vi "Dashboard Main_1366_768.vi"() -> ()   [LabVIEW 2020]
uses:
  <vilib>/Rock Robotics/WPI/ThirdParty/JAS_Junk/TrajLib/TypeDef/FieldDisp_ElementPicture.ctl
  <vilib>/event_ctls.llb/eventvkey.ctl
  <vilib>/Rock Robotics/WPI/ThirdParty/JAS_Junk/TrajLib/Rotation2d_CreateAngle.vi
  <vilib>/Rock Robotics/WPI/ThirdParty/JAS_Junk/TrajLib/Translation2d_Create.vi
  <vilib>/Rock Robotics/WPI/ThirdParty/JAS_Junk/TrajLib/VI/FieldDisp_Element_Rotate.vi
  <vilib>/Rock Robotics/WPI/ThirdParty/JAS_Junk/TrajLib/Conv_Meters_Inches.vi
  <vilib>/Rock Robotics/WPI/ThirdParty/JAS_Junk/TrajLib/Conv_Radians_Deg.vi
  <vilib>/Rock Robotics/WPI/Dashboard/WPI_DashboardLogging Global.vi
  <vilib>/Rock Robotics/Network Tables/NT Read Boolean.vi
  <vilib>/Rock Robotics/Network Tables/NT Write Boolean.vi
  <vilib>/Rock Robotics/Network Tables/NT Read Numeric Array.vi
  <vilib>/picture/pixmap.llb/Flatten Pixmap.vi
  <vilib>/picture/pictutil.llb/Create Mask.vi
  <vilib>/picture/picture.llb/Draw Flattened Pixmap.vi
  <vilib>/Rock Robotics/WPI/ThirdParty/JAS_Junk/TrajLib/Trajectory_Library.lvlib
panel:
  out "Popcorn Engaged":bool
  out "ROBOT":T1
  out "Camera Perf":string
  in  "Camera Settings":T2={"Frame Rate"=30, "Compression"=30, "Size"=1, "DB Camera Config"=FALSE} {"Frame Rate" scale=1.0..30.0; "Compression" scale=100.0..-1.0; "Size" items=["640x480", "320x240", "160x120"]}
  in  "TCP":refnum<k5>
  in  "Rec Mode":enum32{"Stop", "Record", "Playback"}(radio)
  out "Robot IP":string
  out "Image Message":string="Timeout in Camera Communications"
  in  "Dashboard Tab":T3(tab)
  out "MotorChart L":cluster{"Numeric":dbl, "Numeric":dbl}(graph)
  out "MotorSliders L":cluster{"MotorSlide1":dbl, "MotorSlide2":dbl} {"MotorSlide2" scale=-1.0..1.0 scale format="%#_2e"; "MotorSlide1" scale=-1.0..1.0 scale format="%#_2e"}
  out "MotorChart R":cluster{"Numeric":dbl, "Numeric":dbl}(graph)
  out "MotorSliders R":cluster{"MotorSlide1":dbl, "MotorSlide2":dbl} {"MotorSlide2" scale=-1.0..1.0 scale format="%#_2e"; "MotorSlide1" scale=-1.0..1.0 scale format="%#_2e"}
  out "To infinity and beyond?":string
  out "Climb Override":bool
  out "Climbing Stages":sgl(slide) scale=0.0..10.0 scale format="%#_6p"
  out "Reverse":bool
  out "Drive Mode":string
  out "Selected Auto":string
  in  "Select Auto":string(combo)="Select Autonomous ..."
  out "NT Connection":bool
  out "Mode":T4(ring)=enum."Auto Disabled"
  out "Right Camera Perf":cluster{"Bandwidth (Mbps)":dbl, "FPS":dbl}
  in  "ARE YOU READY TO RUMBLE":bool
  out "Lidar":dbl(knob) scale=0.0..10.0
  out "JS2 Z":dbl(slide) scale=-1.0..1.0 scale format="%#_2e"
  out "JS2 Graph":cluster{"X":dbl, "Y":dbl}[](graph)
  out "JS2 Buttons":T5
  out "JS1 Z":dbl(slide) scale=-1.0..1.0 scale format="%#_2e"
  out "JS1 Graph":cluster{"X":dbl, "Y":dbl}[](graph)
  out "JS1 Buttons":T5
  out "Wall!":bool
  out "Right April Tag Updated":bool
  out "Left April Tag Updated":bool
  out "Right Cam Connected":bool
  out "Left Cam Connected":bool
  out "Field Picture":picture
  out "Odom X Pos Ft":dbl format="%14.2f"
  out "Odom Y Pos Ft":dbl format="%14.2f"
  out "Odom Heading Deg":dbl format="%14.2f"
  in  "Shooter Demand":dbl
  out "Shooter Speed":dbl
  out "Shooter Speed Trend":T6(graph)
  out "Target Shooter Speed":dbl
  out "Motor Output":dbl
  in  "Dashboard Tab 2":T7(tab)
  out "Speed Chart Left":cluster{"Numeric":dbl, "Numeric":dbl}(graph)
  out "Speed Chart Right":cluster{"Numeric":dbl, "Numeric":dbl}(graph)
  in  "Dont Question it":bool
  out "Right Speed Demand":dbl
  out "Left Speed Demand":dbl
  out "Right Speed":dbl
  out "Left Speed":dbl
  out "Deviation Threshold 2":dbl
  out "Filter Height 2":dbl
  in  "Deviation Threshold":dbl
  in  "Filter Height":dbl
  out "Current Filter":T8={"Hue"={110.0, 142.0}, "Saturation"={0.0, 209.6394230769231}, "Value"={0.0, 105.16949152542372}} {"Value" scale=0.0..255.0; "Saturation" scale=0.0..255.0; "Hue" scale=0.0..255.0 scale format="%#_3g"}
  in  "New Filter":T8={"Hue"={110.0, 142.0}, "Saturation"={0.0, 209.6394230769231}, "Value"={0.0, 105.16949152542372}} {"Value" scale=0.0..255.0; "Saturation" scale=0.0..255.0; "Hue" scale=0.0..255.0 scale format="%#_3g"}
  in  "Update\nVision\nTuning":bool
  out "Bananas Engaged":bool
  in  "DONUT PRESS":bool
  out "Bandwidth (Mbps)":dbl
  out "FPS":dbl
  in  "Test Slider":dbl(slide) scale=0.0..100.0 scale format="%#_3g"
  in  "On/Off":bool caption="Solenoid"
  in  "Test Name":u16(ring) items=["Select the test to run..."]
  in  "Test Tree":string(tree)
  in  "Motor":cluster{"Value":dbl, "Enable":bool} {"Value" scale=-1.0..1.0 scale format="%#_3g"}
  out "Progress":T9 {"Test Progress" scale=0.0..100.0}
  in  "Rev/Fwd":cluster{"Forward":bool, "Reverse":bool}
  in  "Test Ring":u16(ring) items=["Monochrome", "Color"]
  in  "CheckList":i32(listbox)
  out "Tree":string(tree)
  out "Camera Image":T10(plugin-control)
  out "Background":bool
  in  "Camera Name":string(combo)="No Camera Selection"
  # "HW"
  # "Joysticks"
  # "Drive Motors"
  # "Front"
  # "Left"
  # "Right"
  # "Back"
  # "Right"
  # "Left"
  # "Speed D"
  # "Speed"
  # "DONUT PRESS"
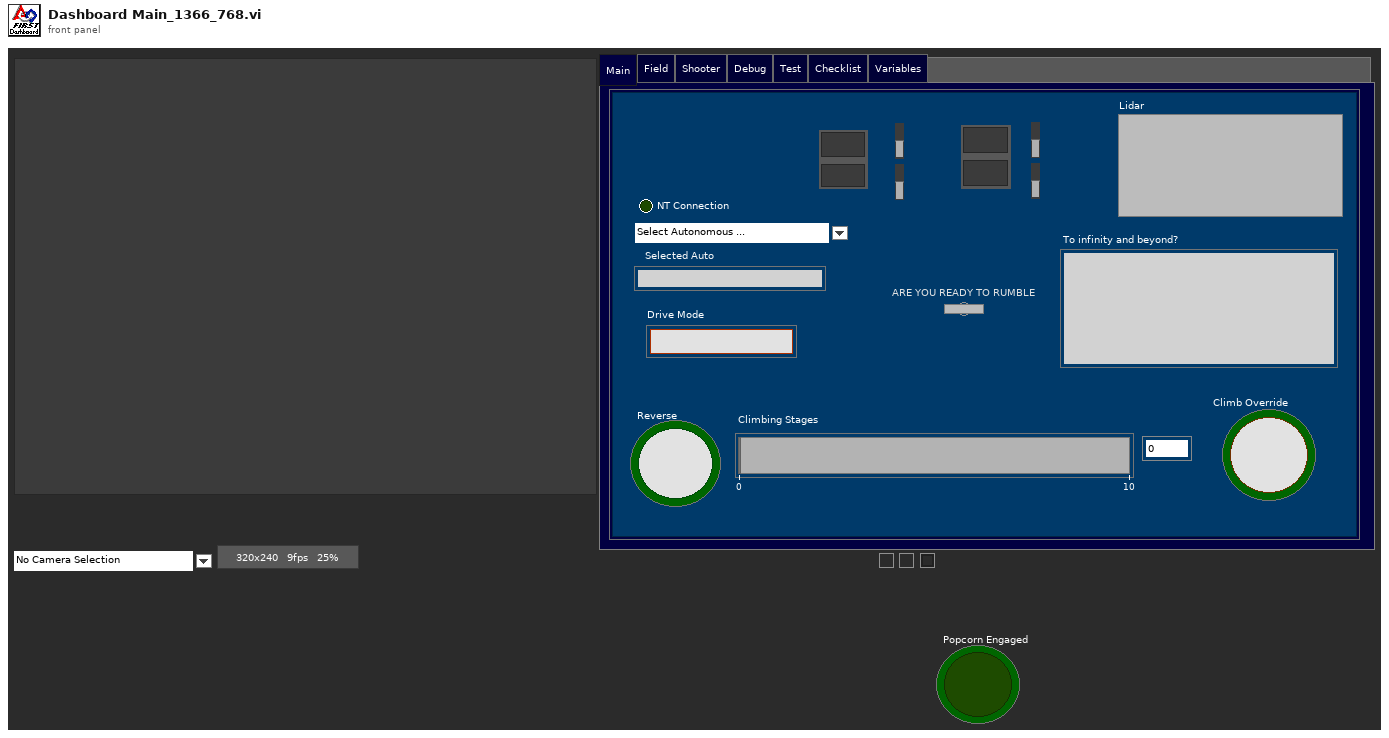
[diagram p1: front panel]
types:
  T1 = typedef "Trajectory_Library.lvlib/FieldDisp_ElementPicture.ctl" = picture
  T2 = cluster{"Frame Rate":i32, "Compression":i32, "Size":u16, "DB Camera Config":bool}
  T3 = enum32{"Main", "Field", "Shooter", "Debug", "Test", "Checklist", "Variables"}
  T4 = enum8{"Tele-Op Disabled", "Tele-Op Enabled", "Auto Disabled", "Auto Enabled", "Test Disabled", "Test Enabled", "Disconnected", "No Code", "E-Stop"}
  T5 = cluster{bool, bool, bool, bool, bool, bool, bool, bool, bool, bool, bool, bool}
  T6 = cluster{"Shooter Demand":dbl, "Numeric":dbl, "Numeric":dbl}
  T7 = enum32{"Drive Left", "Drive Right", "Table", "Camera", "Random"}
  T8 = cluster{"Hue":cluster{dbl, dbl}, "Saturation":cluster{dbl, dbl}, "Value":cluster{dbl, dbl}}
  T9 = cluster{"Test Progress":u8, "Test Progress Text":string}
  T10 = typedef "IMAQ Image.ctl" = refnum<image>
  T11 = cluster{"Save Path":path, "Interval (s)":dbl, "Keep":i32}
  T12 = typedef "Image Type" = u32
  T13 = cluster{"Camera Image":refnum<vi>, "Dashboard Tab":refnum<vi>, "Background":refnum<vi>, "Rec Mode":refnum<vi>, "Test Slider":refnum<vi>, "On/Off ":refnum<vi>, "Test Ring":refnum<vi>, "Rev/Fwd":refnum<vi>, "Test Name":refnum<vi>, "Motor":refnum<vi>, "Progress":refnum<vi>, "CheckList":refnum<vi>, "Tree":refnum<vi>, "Test Tree":refnum<vi>, "Camera Settings":refnum<vi>, "Camera Name":refnum<vi>, "Camera Perf":refnum<vi>}
  T14 = cluster{"Global Rectangle":i32[], "Contours":cluster{"Contour Type":u32, "ROI Type":u32, "Points":i32[]}[]}
  T15 = cluster{"Camera Name":string, string, "Saved DB Images Info":cluster{"Save Path":path, "Interval (s)":dbl, "Keep":i32}}
  T16 = cluster{cluster{dbl, dbl}, cluster{dbl, dbl}, cluster{dbl, dbl}}
  T17 = cluster{"Operation":enum16{"Update", "Clear"}, "Color Box":u32}[]
  T18 = typedef "eventvkey.ctl" = enum16{"ASCII", "Enter", "Return", "Shift", "Ctrl", "Alt", "Cmd", "Opt", "Caps", "NumLock", "Clear", "Break", "Up", "Down", "Left", "Right", "Insert", "Delete", "Home", "End", "PageUp", "PageDown", "Escape", "Help", "Pause", "ScrollLock", "F1", "F2", "F3", "F4", "F5", "F6", "F7", "F8", "F9", "F10", "F11", "F12", "F13", "F14", "F15", "F16", "F17", "F18", "F19", "F20", "F21", "F22", "F23", "F24", "Play", "VolumeUp", "VolumeDown", "Mute", "Two Byte Char"}
  T19 = cluster{"Image Size":bool, "Image Type":bool, "Pixel Value":bool, "ROI Information":bool, "Zoom Factor":bool}
  T20 = cluster{"Operation":enum16{"Update", "Clear"}, "Color Box":u32}
  T21 = cluster{"Shift":bool, "Ctrl":bool, "Alt":bool, "Cmd":bool, "Opt":bool}
  T22 = typedef "Trajectory_Library.lvlib/FieldDisp_FieldElement.ctl" = cluster{"ONE-8-bit pixmap":u8[][], "Two-Array":cdb[][], "Three-Numeric":i32, "Four-Numeric":i32, "Five-Numeric":cdb, "Six-colors":u32[], "Seven-new element/subarray":u32, "Left Poxel":dbl, "Top Pixel":dbl, "Width Pix/Ft":dbl, "Height Pix/Ft":dbl, "Element Picture Ref":refnum<vi>}
  T23 = enum32{"Drive", "Field", "Setup", "Basic", "DrvLeft", "DrvRight", "ArmExtend", "ArmLift", "Bal", "Test", "Checklist", "Variables"}
  T24 = cluster{"Error Strings":string, "Disable Counts":cluster{u16, u16}, "Rail Faults":cluster{u16, u16, u16}, "Robot IP":string, "DB Mode":u8, "Event Info":cluster{"Name":string, "Type":u8, "Number":u16, "Replay":u8}}
  T25 = cluster{"Storage":cluster{"Disk Free":u64, "RAM Block":u32, "RAM free":u32}, "CPU Utilization":cluster{"CPU % ISR":sgl, "CPU % Time Crit":sgl, "CPU % Timed Str":sgl, "CPU % High":sgl, "CPU % Above":sgl, "CPU % Normal":sgl, "CPU % Low":sgl}, "CAN":cluster{"% Bus Utilization":sgl, "Bus Off Cnt":u32, "TX_FIFO Full Cnt":u32, "Receive Error Cnt":u8, "Transmit Error Cnt":u8}, "HID":cluster{"HID Outputs":u32, "Rumble Low":u16, "Rumble High":u16}[]}
  T26 = cluster{"Status bits":cluster{"Test Mode":bool, "Autonomous":bool, "Enabled":bool, "Code Start":bool, "Brownout":bool, "Reserved 2":bool, "Reserved 3":bool, "E-Stop":bool}, "Code Trace":cluster{"Disabled":bool, "TeleOp":bool, "Auto":bool, "Test":bool}, "Controller Type":enum16{"unknown", "cRIO", "roboRio"}, "Code?":enum16{"unknown", "noCode", "code"}, "Battery V":dbl}
  T27 = cluster{"Control Bits":cluster{"TestMode":bool, "Autonomous":bool, "Enabled":bool, "FMS Present":bool, bool, bool, bool, "E-Stop":bool}, "Team Station ":u8, "Countdown":sgl, "Joystick Values":cluster{"Axes":dbl[], "Buttons":bool[], "POVs":i16[]}[]}
  T28 = cluster{"Axes":dbl[], "Buttons":bool[], "POVs":i16[]}[]
  T29 = cluster{"Axes":dbl[], "Buttons":bool[], "POVs":i16[]}
  T30 = cluster{"Buttons[0]":bool, "Buttons[1]":bool, "Buttons[2]":bool, "Buttons[3]":bool, "Buttons[4]":bool, "Buttons[5]":bool, "Buttons[6]":bool, "Buttons[7]":bool, "Buttons[8]":bool, "Buttons[9]":bool, "Buttons[10]":bool, "Buttons[11]":bool}
  T31 = typedef "Trajectory_Library.lvlib/POSE2D.ctl" = cluster{"TRANSLATION":T32, "ROTATION":T33}
  T32 = typedef "Trajectory_Library.lvlib/TRANSLATION2D.ctl" = cluster{"X":dbl, "Y":dbl}
  T33 = typedef "Trajectory_Library.lvlib/ROTATION2D.ctl" = cluster{"VALUE":dbl, "COS":dbl, "SIN":dbl}
  T34 = cluster{"Shooter Demand":dbl, "value":dbl, "value":dbl}
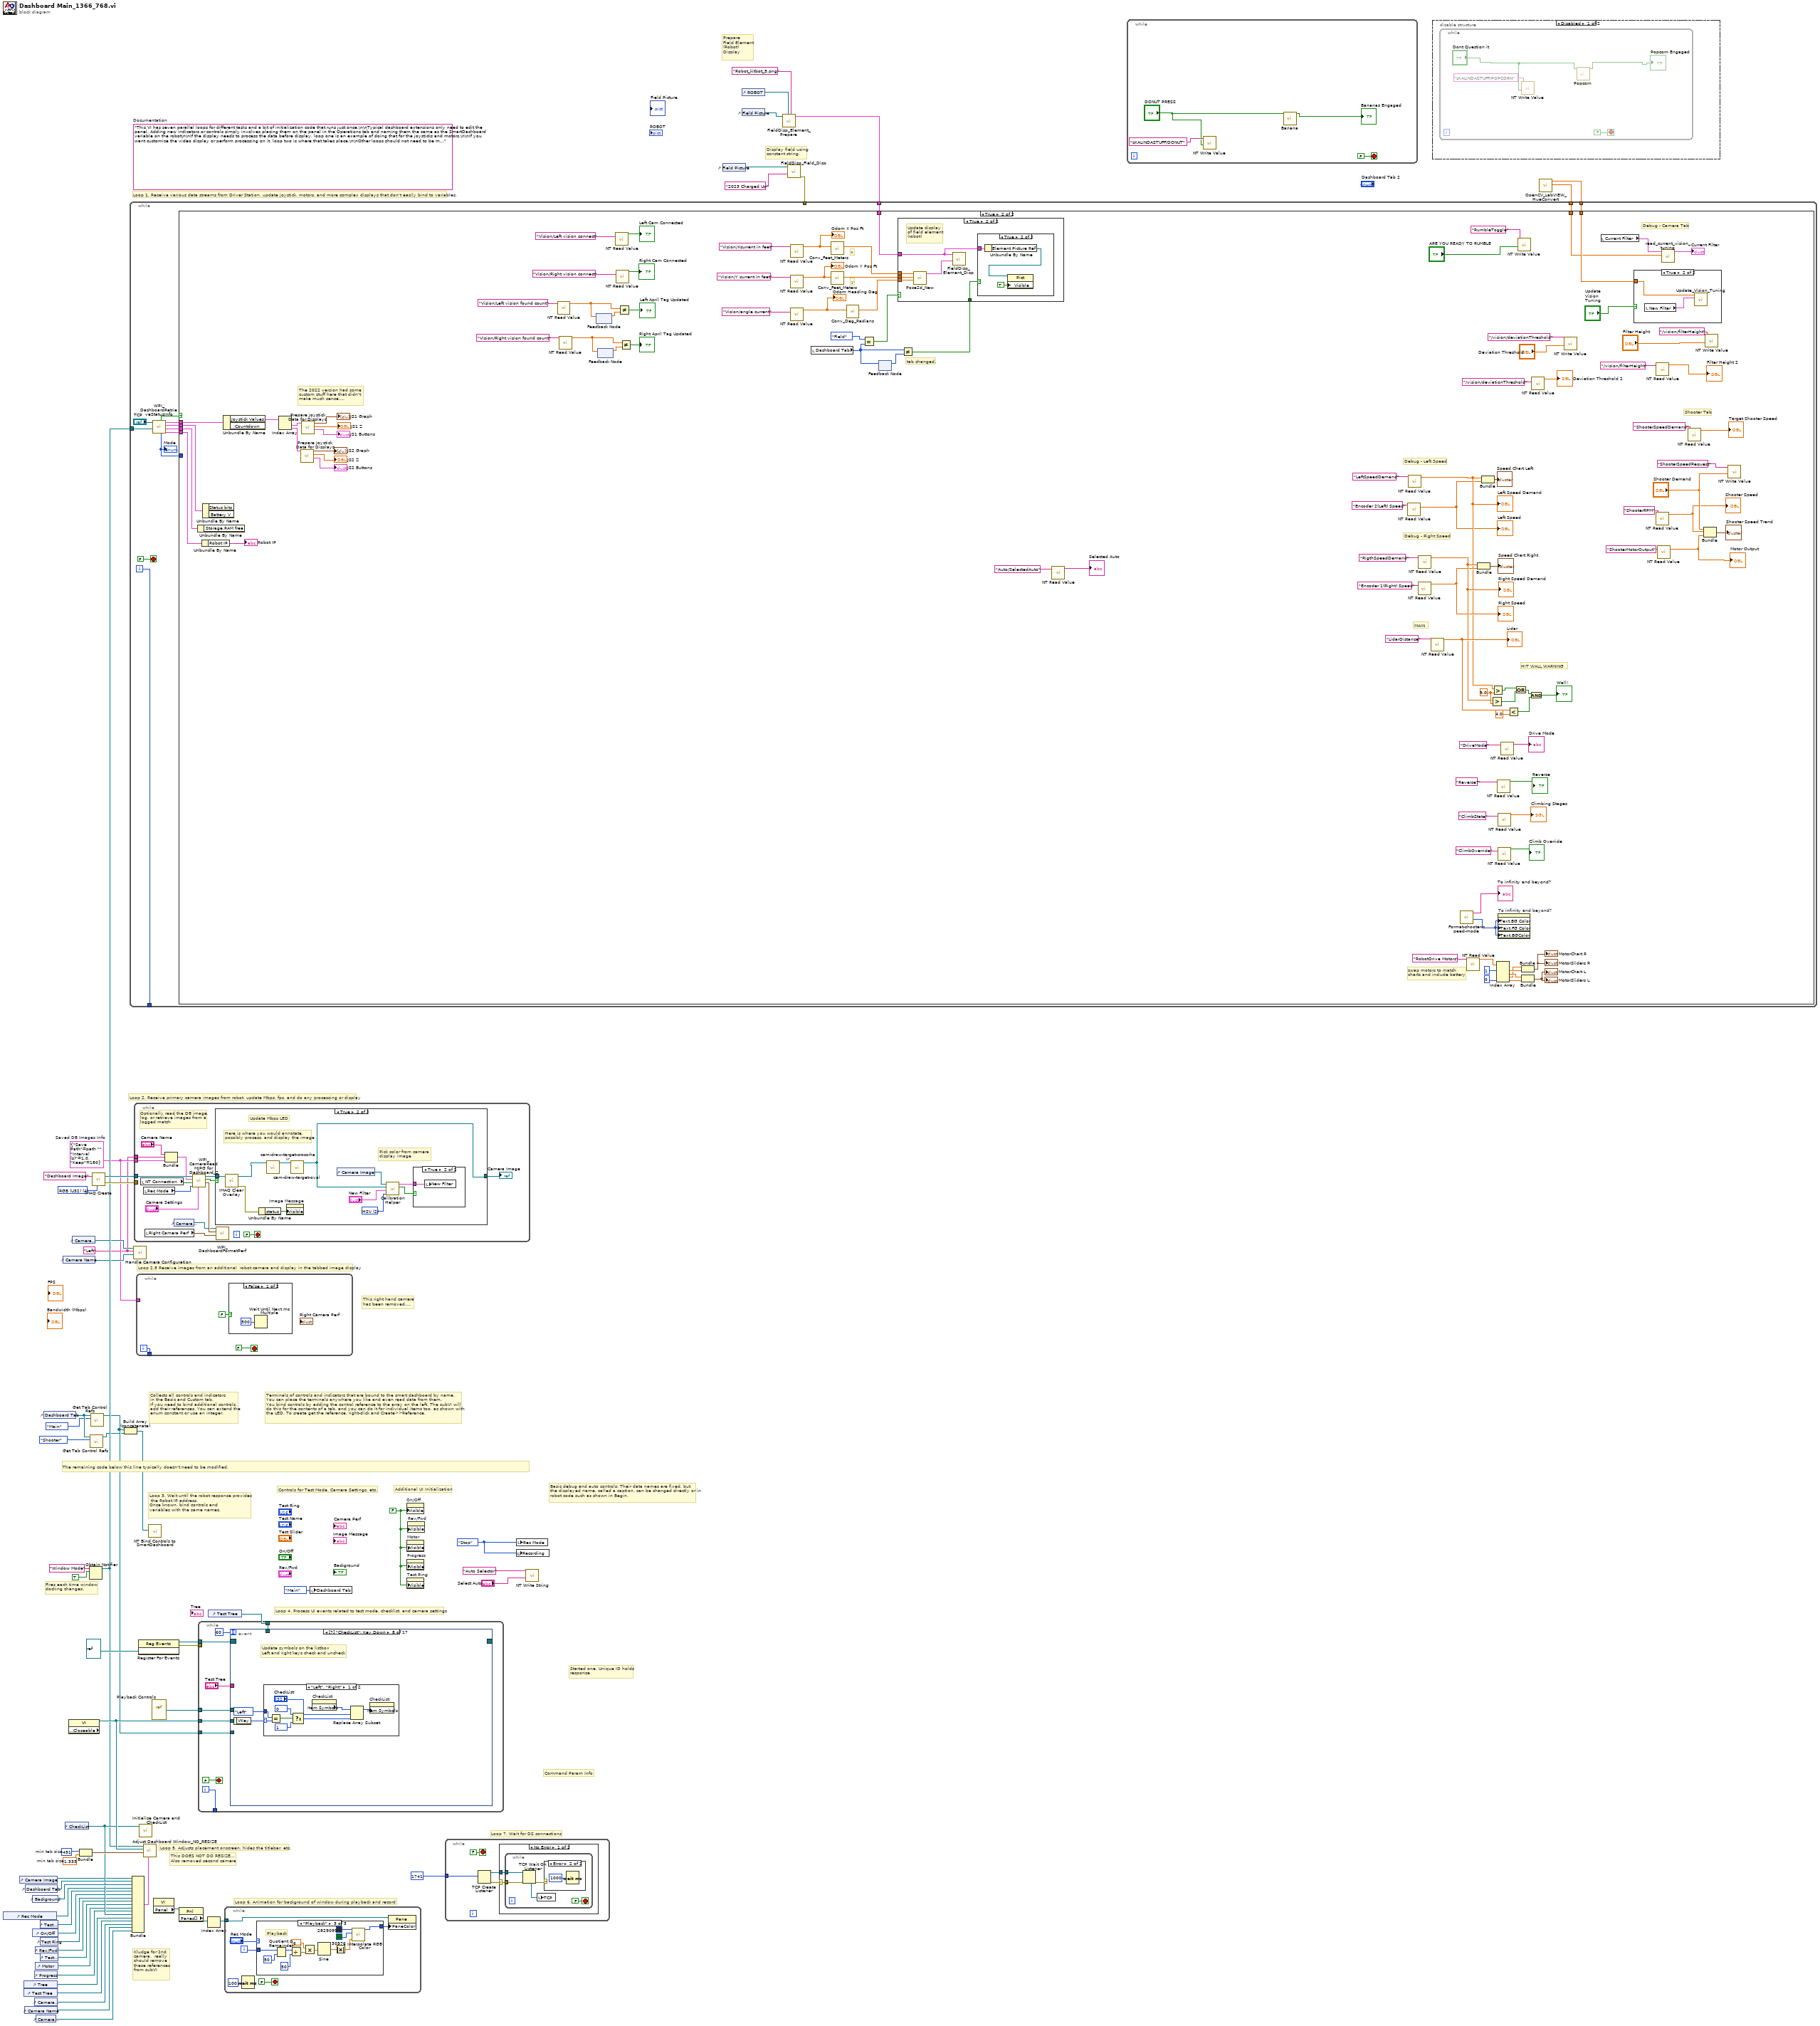
[diagram p0: block diagram]
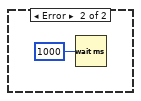
[diagram p5: hidden frame]
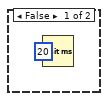
[diagram p6: hidden frame]
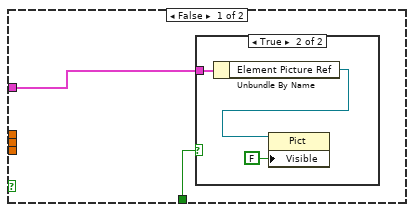
[diagram p8: hidden frame]
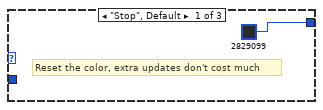
[diagram p11: hidden frame]
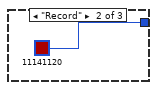
[diagram p12: hidden frame]
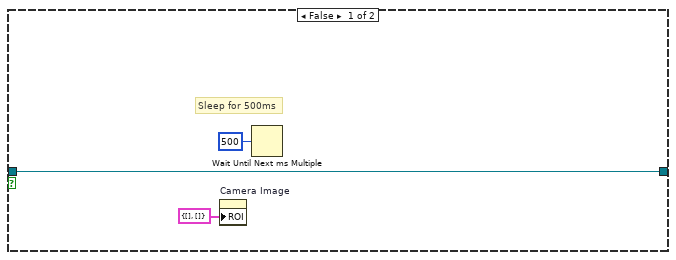
[diagram p13: hidden frame]
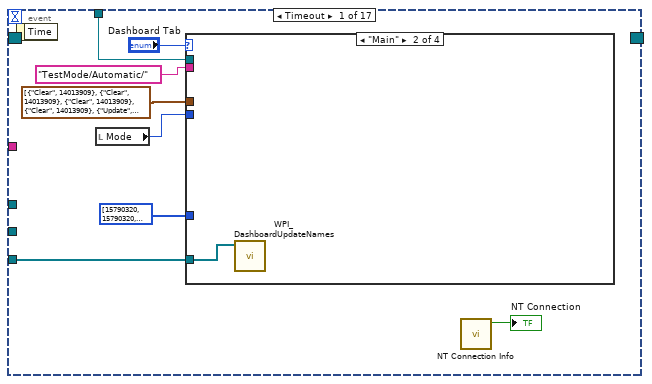
[diagram p15: hidden frame]
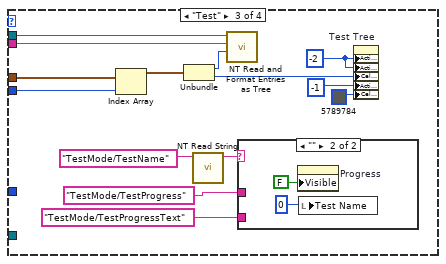
[diagram p17: hidden frame]
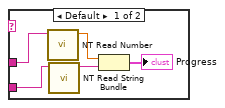
[diagram p18: hidden frame]
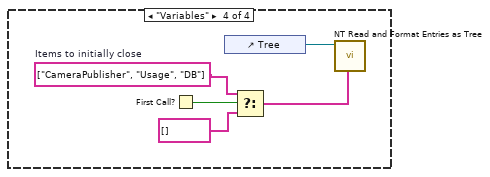
[diagram p19: hidden frame]
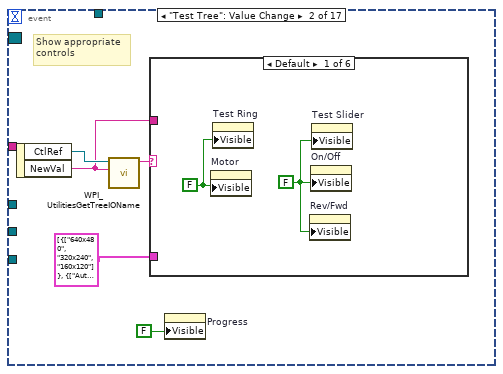
[diagram p20: hidden frame]
diagram:
  w19 = T11 {"Save Path"=path "", "Interval (s)"=1.0, "Keep"=180}  # Saved DB Images Info
  w18 = "Left"
  w44 = 491  # min tab size
  w43 = 1.333  # min tab size
  w48 = enum32{"Stop", "Record", "Playback"}."Stop" ("Rec Mode")
  w28 = FALSE ("Visible")
  (unwired) "This VI has seven parallel loops for different tasks and a bit of initialization code that runs just once.\n\nTypical dashboard extensions only need to edit the panel. Adding new indicators or controls simply involves placing them on the panel in the Operations tab and naming them the same as the SmartDashboard variable on the robot\n\nIf the display needs to process the data before display, loop one is an example of doing that for the joysticks and motors.\n\nIf you want customize the video display or perform processing on it, loop two is where that takes place.\n\nOther loops should not need to be modified. They are pretty standard, and document the task they perform."  # Documentation
  w62 = T12 4 items=["Grayscale (U8)", "Grayscale (I16)", "Grayscale (SGL)", "Complex (CSG)", "RGB (U32)", "HSL (U32)", "RGB (U64)"] ("Image Type")
  # "Display field using\nconstant string."
  # "Prepare\nField Element\n(Robot)\nDisplay"
  # "Kludge for 2nd\ncamera.  really\nshould remove\nthese references\nfrom subVI"
  # "This right hand camera\nhas been removed...."
  # "This DOES NOT DO RESIZE...\nAlso removed second camera"
  # "Loop 2.5 Receive images from an additional  robot camera and display in the tabbed image display"
  # "Command Param Info"
  # "Started one, Unique ID holds\nresponse"
  # "Loop 7. Wait for DS connections"
  # "Basic debug and auto controls: Their data names are fixed, but\nthe displayed name, called a caption, can be changed directly or in\nrobot code such as shown in Begin."
  # "Controls for Test Mode, Camera Settings, etc."
  # "Additional UI Initialization"
  # "Loop 6. Animation for background of window during playback and record"
  # "Fires each time window\ndocking changes."
  # "Collects all controls and indicators\nin the Basic and Custom tab.\nIf you need to bind additional controls,\nadd their references. You can extend the\nenum constant or use an integer."
  # "The remaining code below this line typically doesn't need to be modified."
  # "Loop 4. Process UI events related to test mode, checklist, and camera settings"
  # "Terminals of controls and indicators that are bound to the smart dashboard by name.\nYou can place the terminals anywhere you like and even read data from them.\nYou bind controls by adding the control reference to the array on the left. The subVI will\ndo this for the contents of a tab, and you can do it for individual items too, as shown with\nthe LED. To create get the reference, right-click and Create>>Reference."
  # "Loop 3. Wait until the robot response provides\n the Robot IP address.\nOnce known, bind controls and\nvariables with the same names."
  # "Loop 5. Adjusts placement onscreen, hides the titlebar, etc."
  # "Loop 1. Receive various data streams from Driver Station, update joystick, motors, and more complex displays that don't easily bind to variables."
  # "Loop 2. Receive primary camera images from robot, update Mbps, fps, and do any processing or display"
  n1 = control-ref of="Rec Mode"() -> (w34:refnum<vi>)
  n2 = control-ref of="Camera Image"() -> (w15:refnum<vi>)
  n3 = control-ref of="Tree"() -> (w38:refnum<vi>)
  n4 = control-ref of="Test Tree"() -> (w37:refnum<vi>)
  n5 = control-ref of="Camera Name"() -> (w16:refnum<vi>)
  n6 = control-ref of="Dashboard Tab"() -> (w45:refnum<vi>)
  n7 = control-ref of="Background"() -> (w41:refnum<vi>)
  n8 = control-ref of="On/Off"() -> (w32:refnum<vi>)
  n9 = control-ref of="Progress"() -> (w29:refnum<vi>)
  n10 = control-ref of="Camera Settings"() -> (w17:refnum<vi>)
  n11 = control-ref of="Rev/Fwd"() -> (w30:refnum<vi>)
  n12 = control-ref of="Motor"() -> (w35:refnum<vi>)
  n13 = control-ref of="Camera Perf"() -> (w23:refnum<vi>)
  n14 = control-ref of="Test Slider"() -> (w33:refnum<vi>)
  n15 = control-ref of="Test Ring"() -> (w31:refnum<vi>)
  n16 = control-ref of="Test Name"() -> (w36:refnum<vi>)
  n17 = control-ref of="Dashboard Tab"() -> (w7:refnum<vi>)
  n18 = control-ref of="Camera Name"() -> (w24:refnum<vi>)
  n19 = control-ref of="CheckList"() -> (w39:refnum<vi>)
  n20 = property class="VI" props=["Front Panel.Closeable"]() -> (reference out=w47:refnum<vi>)  [unwired: 2 in, 2 out]
  n21 = control-ref of="Camera Settings"() -> (w25:refnum<vi>)
  n22 = Bundle("min tab size"=w44, "min tab size"=w43) -> (w42:cluster{"min tab size":i32, "min tab size":dbl})  [unwired: 1 in]
  n23 = Obtain Notifier(name (unnamed)="Window Mode", notification data type=TRUE) -> (notifier out=w27:refnum<notifier>)  [unwired: 2 in, 2 out]
  n24 = call <vilib>:"Get Tab Control Refs.vi"("Page Index"=T3."Shooter" ("Dashboard Tab"), "TabControl in"=w7) -> ("ControlsOnPage"=w8:refnum<vi>[])  [unwired: 9 in]
  n25 = call <vilib>:"Get Tab Control Refs.vi"("Page Index"=T3."Main" ("Dashboard Tab"), "TabControl in"=w7) -> ("ControlsOnPage"=w22:refnum<vi>[])  [unwired: 9 in]
  n26 = call "IMAQ Create"("Image Name"="Dashboard Image", "Image Type"=w62) -> ("New Image"=w60:T10, "error out"=w59:errorcluster)  [unwired: 2 in, 1 out]
  n27 = Build Array (concatenate)(w22, w8) -> (w46:refnum<vi>[])
  n28 = Bundle("Camera Image"=w15, "Dashboard Tab"=w45, "Background"=w41, "Rec Mode"=w34, "Test Slider"=w33, "On/Off"=w32, "Test Ring"=w31, "Rev/Fwd"=w30, "Test Name"=w36, "Motor"=w35, "Progress"=w29, "CheckList"=w39, "Tree"=w38, "Test Tree"=w37, "Camera Settings"=w17, "Camera Name"=w16, "Camera Perf"=w23) -> (w40:T13)  [unwired: 1 in]
  n29 = call "Handle Camera Configuration.vi"("CameraNameRef"=w24, "Display Name"=w18, "ClusterRef"=w25) -> ()  [unwired: 9 in]
  n30 = while {
    tunnel: w60 -> [w76]
    tunnel: w59 -> [_]
    tunnel: w19 -> [w69]
    tunnel: w18 -> [w66]
    stop <- FALSE stop-if-true
    # "Optionally read the DB image,\nlog, or retrieve images from a\nlogged match"
    n31 = local read "NT Connection"() -> (w70:bool)
    n32 = local read "Rec Mode"() -> (w73:enum32{"Stop", "Record", "Playback"})
    n33 = local read "Right Camera Perf"() -> (w64:cluster{"Bandwidth (Mbps)":dbl, "FPS":dbl})
    n34 = Bundle("Camera Name"="Camera Name", w66, "Saved DB Images Info"=w69) -> (w68:T15)  [unwired: 1 in]
    n35 = control-ref of="Camera Perf"() -> (w63:refnum<vi>)
    n36 = call <vilib>:"WPI_CameraRead MJPG for Dashboard_2.vi"("Camera Settings"="Camera Settings", "Rec Mode"=w73, "NT Connection"=w70, "Capture Info"=w68, "Image in"=w76) -> ("perf info"=w65:cluster{"Bandwidth (Mbps)":dbl, "fps":dbl}, "Active"=w74:bool, "Image\\ out"=w75:T10)  [unwired: 4 in]
    n37 = case shown="True" w74 {
      tunnel: w75 -> [w79 w89]
      tunnel: [w79 w83] -> w71
      frame False {
        # "Sleep for 500ms"
        n38 = property on="Camera Image" class="ImageControl"("ROI"=T14 {"Global Rectangle"=[], "Contours"=[]}) -> ()  [unwired: 2 in, 2 out]
        n39 = Wait Until Next ms Multiple(millisecond multiple=u32 500) -> ()  [unwired: 1 out]
      }
      frame True {
        w84 = u16 2 items=["RGB", "HSL", "HSV", "HSI", "CIE L*a*b*", "CIE XYZ"] ("Color Mode")
        # "Pick color from camera\ndisplay image"
        # "Here is where you would annotate,\npossibly process, and display the image"
        # "Update Mbps LED"
        n40 = call "IMAQ Clear Overlay"("Image"=w89) -> ("error out"=w90:errorcluster, "Image Out"=w88:T10)  [unwired: 2 in, 7 out]
        n41 = Unbundle By Name(w90) -> ("status"=w91:bool)
        n42 = call "cam-draw-target-cross-hair.vi"("Refnum in"=w88) -> ("Refnum out"=w87:T10)  [unwired: 10 in]
        n43 = property on="Image Message" class="Str"("Visible"=w91) -> ()  [unwired: 2 in, 2 out]
        n44 = call "cam-draw-target-oval.vi"("Refnum in"=w87) -> ("Refnum out"=w83:T10)  [unwired: 10 in]
        n45 = control-ref of="Camera Image"() -> (w82:refnum<vi>)
        n46 = call "Calibration Helper.vi"("Color Mode"=w84, "Color Components"="New Filter", "Image"=w83, "Image Ctl Refnum"=w82) -> ("Changed"=w86:bool, "output color"=w85:T16)  [unwired: 6 in]
        n47 = case shown="True" w86 {
          tunnel: w85 -> [_ w92]
          frame False {
          }
          frame True {
            n48 = local write "New Filter"(w92) -> ()
          }
        }
      }
    }
    "Camera Image" <- w71
    n49 = call <vilib>:"WPI_DashboardFormatPerf.vi"("Right Camera Perf"=w64, "Performance"=w65, "String in"=w63) -> ()  [unwired: 9 in]
  }
  n50 = while {
    tunnel: [w94] -> _
    tunnel: w19 -> [_]
    i -> [w94]
    stop <- FALSE stop-if-true
    n51 = case shown="False" FALSE {
      frame False {
        n52 = Wait Until Next ms Multiple(millisecond multiple=u32 500) -> ()  [unwired: 1 out]
      }
      frame True {
      }
    }
  }
  n53 = register-events(refnum<vi> refnum) -> (reference out=w51:refnum<event-registration>, error out=w50:errorcluster)  [unwired: 2 in]
  n54 = call "Initialize Camera and CheckList.vi"("ListBox in"=w39) -> ()  [unwired: 11 in]
  n55 = call "Adjust Dashboard Window_NO_RESIZE.vi"("Sizing Refnums"=w40, "Size Constraints"=w42, "VI"=w47, "WIn Mode"=w27) -> ()  [unwired: 8 in]
  n56 = call <vilib>:"NT Bind Controls to SmartDashboard.vi"("Bound Control Refs"=w46) -> ()  [unwired: 11 in]
  n57 = vi-ref "Playback Controls.vi"() -> (w52:refnum<vi>)
  n58 = property class="VI"() -> ("Panel"=w54:refnum<vi>)  [unwired: 2 in, 2 out]
  n59 = property class="Pnl"(reference=w54) -> ("Panes[]"=w55:refnum<vi>[])  [unwired: 1 in, 2 out]
  n60 = Index Array(array=w55) -> (element=w53:refnum<vi>)  [unwired: 1 in]
  n61 = control-ref of="Test Tree"() -> (w56:refnum<vi>)
  n62 = while {
    tunnel: [w102] -> _
    tunnel: w56 -> [w101]
    tunnel: w52 -> [w100]
    tunnel: w51 -> [w99]
    tunnel: w50 -> [_]
    tunnel: w47 -> [w98]
    tunnel: w22 -> [w97]
    i -> [w102]
    stop <- FALSE stop-if-true
    n63 = event shown="[7] \"CheckList\": Key Down" {
      selector: w99 -> [_ _ _ _ _ _ _ _ _ _ _ _ _ _ _ _ _]
      dyn-events: [_ _ _ _ _ _ _ _ _ _ _ _ _ w307 _ _ _] -> _
      timeout: u32 60 ("milliseconds to wait") -> [_ _ _ _ _ _ _ _ _ _ _ _ _ _ _ _ _]
      tunnel: w101 -> [w112 _ _ _ _ _ _ _ _ _ _ _ _ _ _ _ _]
      tunnel: "Test Tree" -> [_ _ _ _ _ _ _ _ w280 w287 w288 w291 w298 _ _ _ _]
      tunnel: w100 -> [_ _ _ _ _ _ _ _ _ _ _ _ _ w309 _ w324 _]
      tunnel: w98 -> [_ _ _ _ _ _ _ _ _ _ _ _ _ w305 _ _ _]
      tunnel: w97 -> [w107 _ _ _ _ _ _ _ _ _ _ _ _ _ _ _ _]
      event Timeout {
        n64 = event-data() -> ()  [unwired: 1 in, 1 out]
        n65 = local read "Mode"() -> (w110:T4)
        n66 = case shown="\"Main\"" "Dashboard Tab" {
          tunnel: w112 -> [_ _ w128 _]
          tunnel: "TestMode/Automatic/" ("Name Pattern") -> [_ _ w127 _]
          tunnel: T17 [{"Operation"=enum."Clear", "Color Box"=14013909}, {"Operation"=enum."Clear", "Color Box"=14013909}, {"Operation"=enum."Clear", "Color Box"=14013909}, {"Operation"=enum."Clear", "Color Box"=14013909}, {"Operation"=enum."Update", "Color Box"=14013909}, {"Operation"=enum."Update", "Color Box"=16777215}, {"Operation"=enum."Clear", "Color Box"=14013909}, {"Operation"=enum."Clear", "Color Box"=14013909}, {"Operation"=enum."Clear", "Color Box"=14013909}] -> [_ _ w120 _]
          tunnel: w110 -> [_ _ w119 _]
          tunnel: u32[] [15790320, 15790320, 15790320, 15790320, 16777215, 16777215, 15790320, 15790320, 15790320] -> [_ _ _ _]
          tunnel: w107 -> [_ w114 _ _]
          frame Default {
          }
          frame "Main" {
            n67 = call <vilib>:"WPI_DashboardUpdateNames.vi"("Controls on Tab"=w114) -> ()  [unwired: 11 in]
          }
          frame "Test" {
            w126 = -2 ("Active Item:Row Number")
            n68 = Index Array(array=w120, index=w119) -> (element=w121:T20)
            n69 = Unbundle(w121) -> ("Operation"=w122:enum16{"Update", "Clear"}, "Color Box"=w123:u32)
            n70 = call <vilib>:"NT Read String.vi"("name"="TestMode/TestName" ("Name")) -> ("value"=w117:string)  [unwired: 8 in, 2 out]
            n71 = call <vilib>:"NT Read and Format Entries as Tree.vi"("Operation"=w122, "Name Pattern"=w127, "Tree Refnum"=w128) -> ()  [unwired: 7 in, 2 out]
            n72 = case shown="\"\"" w117 {
              tunnel: "TestMode/TestProgress" ("Name") -> [w130 _]
              tunnel: "TestMode/TestProgressText" ("Name") -> [w129 _]
              frame Default {
                n73 = call <vilib>:"NT Read Number.vi"("name"=w130) -> ("value"=w131:dbl)  [unwired: 8 in, 2 out]
                n74 = call <vilib>:"NT Read String.vi"("name"=w129) -> ("value"=w132:string)  [unwired: 8 in, 2 out]
                n75 = Bundle("value"=w131, "value"=w132) -> (→"Progress":cluster{"value":dbl, "value":string})  [unwired: 1 in]
              }
              frame "" {
                n76 = property on="Progress" class="Clust (strict)"("Visible"=FALSE) -> ()  [unwired: 2 in, 2 out]
                n77 = local write "Test Name"(u16 0) -> ()
              }
            }
            n78 = property on="Test Tree" class="Tree (strict)"("Active Item Row Number"=w126, "ActiveColNum"=w126, "CellBG"=w123, "Active Item Row Number"=-1 ("Active Item:Row Number"), "CellBG"=u32 5789784 ("Color Box")) -> ()  [unwired: 2 in, 2 out]
          }
          frame "Variables" {
            w138 = string[] ["CameraPublisher", "Usage", "DB"]  # Items to initially close
            n79 = First Call?() -> (First Call?: T/F=w139:bool)
            n80 = control-ref of="Tree"() -> (w140:refnum<vi>)
            n81 = Select(t=w138, s=w139, f=string[] []) -> (s? t:f=w136:string[])
            n82 = call <vilib>:"NT Read and Format Entries as Tree.vi"("Tags to  Close"=w136, "Tree Refnum"=w140) -> ()  [unwired: 8 in, 2 out]
          }
        }
        n83 = call <vilib>:"NT Connection Info.vi"() -> ("Connected"=→"NT Connection":bool)  [unwired: 11 in]
      }
      event "Test Tree": Value Change {
        # "Show appropriate\ncontrols"
        n84 = event-data() -> ("CtlRef"=w144:refnum<vi>, "NewVal"=w142:string)  [unwired: 1 in]
        n85 = call <vilib>:"WPI_UtilitiesGetTreeIOName.vi"("NewVal"=w142, "TreeControl in"=w144) -> ("I/O Name"=w145:string)  [unwired: 9 in]
        n86 = case shown="Default" w145 {
          selector: w145 -> [_ w152 _ w174 w183 _]
          tunnel: w142 -> [_ _ w171 w173 _ w190]
          tunnel: cluster{string[]}[] [{["640x480", "320x240", "160x120"]}, {["Auto", "Fixed indoor", "Fixed outdoor 1", "Fixed outdoor 2", "Fixed fluorescent 1", "Fixed fluorescent 2", "Hold current"]}, {["Auto", "Flicker-free 50 Hz", "Flicker-free 60 Hz", "Hold current"]}, {["None", "Prioritize frame rate", "Prioritize image quality"]}, {["Monochrome", "Color"]}] -> [_ _ _ _ _ w189]
          frame Default {
            w147 = FALSE ("Visible")
            w146 = FALSE ("Visible")
            n87 = property on="Motor" class="Clust (strict)"("Visible"=w146) -> ()  [unwired: 2 in, 2 out]
            n88 = property on="Test Ring" class="Ring (strict)"("Visible"=w146) -> ()  [unwired: 2 in, 2 out]
            n89 = property on="Rev/Fwd" class="Clust (strict)"("Visible"=w147) -> ()  [unwired: 2 in, 2 out]
            n90 = property on="On/Off" class="Bool (strict)"("Visible"=w147) -> ()  [unwired: 2 in, 2 out]
            n91 = property on="Test Slider" class="Slide (strict)"("Visible"=w147) -> ()  [unwired: 2 in, 2 out]
          }
          frame "Analog Out", "Motor", "PWM" {
            w153 = FALSE ("Visible")
            n92 = case shown="\"Analog Out\"" w152 {
              tunnel: [1.0 ("Value") -1.0 ("Value") 0.0 ("Value")] -> w151
              tunnel: [255.0 ("Value") 1.0 ("Value") 5.0 ("Value")] -> w150
              tunnel: [128.0 ("Value") 0.0 ("Value") 0.0 ("Value")] -> w149
              tunnel: [64.0 ("Value") 0.5 ("Value") 1.0 ("Value")] -> w148
              frame "PWM" {
              }
              frame "Motor", Default {
              }
              frame "Analog Out" {
              }
            }
            n93 = property on="Motor" class="Clust (strict)"("Visible"=TRUE) -> ()  [unwired: 2 in, 2 out]
            n94 = property on="Value" class="Slide (strict)"("Value"=w149, "Scale.Minimum"=w151, "Scale.Maximum"=w150, "Scale.Increment"=w148) -> ()  [unwired: 2 in, 2 out]
            n95 = property on="On/Off" class="Bool (strict)"("Visible"=w153) -> ()  [unwired: 2 in, 2 out]
            n96 = property on="Test Slider" class="Slide (strict)"("Visible"=w153) -> ()  [unwired: 2 in, 2 out]
            n97 = property on="Test Ring" class="Ring (strict)"("Visible"=w153) -> ()  [unwired: 2 in, 2 out]
            n98 = property on="Rev/Fwd" class="Clust (strict)"("Visible"=w153) -> ()  [unwired: 2 in, 2 out]
          }
          frame "Servo" {
            w169 = FALSE ("Visible")
            n99 = call <vilib>:"NT Read Number.vi"("name"=w171) -> ("value"=w170:dbl)  [unwired: 8 in, 2 out]
            n100 = property on="Test Slider" class="Slide (strict)"("Visible"=TRUE, "Scale.Maximum"=170.0 ("Scale.Range:Maximum")) -> ()  [unwired: 2 in, 2 out]
            n101 = local write "Test Slider"(w170) -> ()
            n102 = property on="Motor" class="Clust (strict)"("Visible"=w169) -> ()  [unwired: 2 in, 2 out]
            n103 = property on="Rev/Fwd" class="Clust (strict)"("Visible"=w169) -> ()  [unwired: 2 in, 2 out]
            n104 = property on="On/Off" class="Bool (strict)"("Visible"=w169) -> ()  [unwired: 2 in, 2 out]
            n105 = property on="Test Ring" class="Ring (strict)"("Visible"=w169) -> ()  [unwired: 2 in, 2 out]
          }
          frame "Relay", "Solenoid" {
            w172 = FALSE ("Visible")
            n106 = property on="Motor" class="Clust (strict)"("Visible"=w172) -> ()  [unwired: 2 in, 2 out]
            n107 = property on="Test Slider" class="Slide (strict)"("Visible"=w172) -> ()  [unwired: 2 in, 2 out]
            n108 = Search and Replace String(input string=w173, search string="/Value  **", replace string="/Direction") -> (result string=w179:string)  [unwired: 5 in, 3 out]
            n109 = property on="Test Ring" class="Ring (strict)"("Visible"=w172) -> ()  [unwired: 2 in, 2 out]
            n110 = call <vilib>:"NT Read String.vi"("name"=w179) -> ("value"=w177:string)  [unwired: 8 in, 2 out]
            n111 = Equal?(x="Both directions", y=w177) -> (x = y?=w175:bool)
            n112 = Not(x=w175) -> (.not. x?=w176:bool)
            n113 = property on="Rev/Fwd" class="Clust (strict)"("Visible"=w175) -> ()  [unwired: 2 in, 2 out]
            n114 = property on="On/Off" class="Bool (strict)"("Visible"=w176, "Caption.Text"=w174) -> ()  [unwired: 2 in, 2 out]
          }
          frame "Compressor", "Digital Out" {
            w182 = FALSE ("Visible")
            # "Get direction and finish"
            n115 = property on="Motor" class="Clust (strict)"("Visible"=w182) -> ()  [unwired: 2 in, 2 out]
            n116 = property on="Test Slider" class="Slide (strict)"("Visible"=w182) -> ()  [unwired: 2 in, 2 out]
            n117 = property on="Test Ring" class="Ring (strict)"("Visible"=w182) -> ()  [unwired: 2 in, 2 out]
            n118 = property on="On/Off" class="Bool (strict)"("Visible"=TRUE, "Caption.Text"=w183) -> ()  [unwired: 2 in, 2 out]
            n119 = property on="Rev/Fwd" class="Clust (strict)"("Visible"=FALSE) -> ()  [unwired: 2 in, 2 out]
          }
          frame "Camera" {
            n120 = call <vilib>:"NT_Get Last Path Segment.vi"("String in"=w190) -> ("String out"=w191:string)  [unwired: 10 in]
            n121 = property on="On/Off" class="Bool (strict)"("Visible"=FALSE) -> ()  [unwired: 2 in, 2 out]
            n122 = property on="Motor" class="Clust (strict)"("Visible"=FALSE) -> ()  [unwired: 2 in, 2 out]
            n123 = property on="Rev/Fwd" class="Clust (strict)"("Visible"=FALSE) -> ()  [unwired: 2 in, 2 out]
            n124 = case shown="\"White Balance  **\"" w191 {
              tunnel: w190 -> [w197 w206 w215 w224 w233 _ w239]
              tunnel: w189 -> [w195 w203 w212 w221 w230 _ _]
              frame "Size  **" {
                n125 = Index Array(array=w195) -> (element=w194:cluster{string[]})  [unwired: 1 in]
                n126 = call <vilib>:"NT Read String.vi"("name"=w197) -> ("value"=w196:string)  [unwired: 8 in, 2 out]
                n127 = Unbundle(w194) -> (w192:string[])
                n128 = Match First String(2:w192, 3:w196) -> (0:w193:i32)  [unwired: 1 out]
                n129 = property on="Test Ring" class="Ring (strict)"("Value"=w193, "Strings []"=w192) -> ()  [unwired: 2 in, 2 out]
                n130 = property on="Test Ring" class="Ring (strict)"("Visible"=TRUE) -> ()  [unwired: 2 in, 2 out]
                n131 = property on="Test Slider" class="Slide (strict)"("Visible"=FALSE) -> ()  [unwired: 2 in, 2 out]
              }
              frame "White Balance  **" {
                n132 = Index Array(array=w203, index=1) -> (element=w204:cluster{string[]})
                n133 = call <vilib>:"NT Read String.vi"("name"=w206) -> ("value"=w205:string)  [unwired: 8 in, 2 out]
                n134 = Unbundle(w204) -> (w201:string[])
                n135 = Match First String(2:w201, 3:w205) -> (0:w200:i32)  [unwired: 1 out]
                n136 = property on="Test Ring" class="Ring (strict)"("Value"=w200, "Strings []"=w201) -> ()  [unwired: 2 in, 2 out]
                n137 = property on="Test Ring" class="Ring (strict)"("Visible"=TRUE) -> ()  [unwired: 2 in, 2 out]
                n138 = property on="Test Slider" class="Slide (strict)"("Visible"=FALSE) -> ()  [unwired: 2 in, 2 out]
              }
              frame "Exposure  **" {
                n139 = Index Array(array=w212, index=2) -> (element=w213:cluster{string[]})
                n140 = call <vilib>:"NT Read String.vi"("name"=w215) -> ("value"=w214:string)  [unwired: 8 in, 2 out]
                n141 = Unbundle(w213) -> (w209:string[])
                n142 = Match First String(2:w209, 3:w214) -> (0:w210:i32)  [unwired: 1 out]
                n143 = property on="Test Ring" class="Ring (strict)"("Value"=w210, "Strings []"=w209) -> ()  [unwired: 2 in, 2 out]
                n144 = property on="Test Ring" class="Ring (strict)"("Visible"=TRUE) -> ()  [unwired: 2 in, 2 out]
                n145 = property on="Test Slider" class="Slide (strict)"("Visible"=FALSE) -> ()  [unwired: 2 in, 2 out]
              }
              frame "Exposure Priority  **" {
                n146 = Index Array(array=w221, index=3) -> (element=w222:cluster{string[]})
                n147 = call <vilib>:"NT Read String.vi"("name"=w224) -> ("value"=w223:string)  [unwired: 8 in, 2 out]
                n148 = Unbundle(w222) -> (w218:string[])
                n149 = Match First String(2:w218, 3:w223) -> (0:w219:i32)  [unwired: 1 out]
                n150 = property on="Test Ring" class="Ring (strict)"("Value"=w219, "Strings []"=w218) -> ()  [unwired: 2 in, 2 out]
                n151 = property on="Test Ring" class="Ring (strict)"("Visible"=TRUE) -> ()  [unwired: 2 in, 2 out]
                n152 = property on="Test Slider" class="Slide (strict)"("Visible"=FALSE) -> ()  [unwired: 2 in, 2 out]
              }
              frame "Color Enable  **" {
                n153 = Index Array(array=w230, index=4) -> (element=w231:cluster{string[]})
                n154 = call <vilib>:"NT Read String.vi"("name"=w233) -> ("value"=w232:string)  [unwired: 8 in, 2 out]
                n155 = Unbundle(w231) -> (w227:string[])
                n156 = Match First String(2:w227, 3:w232) -> (0:w228:i32)  [unwired: 1 out]
                n157 = property on="Test Ring" class="Ring (strict)"("Value"=w228, "Strings []"=w227) -> ()  [unwired: 2 in, 2 out]
                n158 = property on="Test Ring" class="Ring (strict)"("Visible"=TRUE) -> ()  [unwired: 2 in, 2 out]
                n159 = property on="Test Slider" class="Slide (strict)"("Visible"=FALSE) -> ()  [unwired: 2 in, 2 out]
              }
              frame Default {
                n160 = property on="Test Ring" class="Ring (strict)"("Visible"=FALSE) -> ()  [unwired: 2 in, 2 out]
                n161 = property on="Test Slider" class="Slide (strict)"("Visible"=FALSE) -> ()  [unwired: 2 in, 2 out]
              }
              frame "Brightness  **", "Color Level  **", "Compression  **", "FPS  **", "Sharpness  **" {
                n162 = call <vilib>:"NT Read Number.vi"("name"=w239) -> ("value"=w238:dbl)  [unwired: 8 in, 2 out]
                n163 = local write "Test Slider"(w238) -> ()
                n164 = property on="Test Slider" class="Slide (strict)"("Visible"=TRUE, "Scale.Maximum"=100.0 ("Scale.Range:Maximum")) -> ()  [unwired: 2 in, 2 out]
                n165 = property on="Test Ring" class="Ring (strict)"("Visible"=FALSE) -> ()  [unwired: 2 in, 2 out]
              }
            }
          }
        }
        n166 = property on="Progress" class="Clust (strict)"("Visible"=FALSE) -> ()  [unwired: 2 in, 2 out]
      }
      event "Test Name": Mouse Enter {
        # "Populate the ring with the list of tests"
        n167 = event-data() -> ()  [unwired: 1 in, 1 out]
        n168 = call <vilib>:"NT Read String Array.vi"("name"="TestMode/TestList" ("Name")) -> ("value"=w246:string[])  [unwired: 8 in, 2 out]
        n169 = Build Array (concatenate)("Select the test to run...", w246) -> (w245:string[])
        n170 = property on="Test Name" class="Ring (strict)"("Strings []"=w245) -> ()  [unwired: 2 in, 2 out]
      }
      event "Test Name": Value Change {
        w247 = FALSE ("Visible")
        # "Tell the robot the test name to run"
        n171 = event-data() -> ("NewVal"=w251:u16)  [unwired: 1 in]
        n172 = property on="Test Name" class="Ring (strict)"() -> ("Strings []"=w252:string[])  [unwired: 2 in, 2 out]
        n173 = local write "Progress"(T9 {"Test Progress"=0, "Test Progress Text"=""} ("Progress")) -> ()
        n174 = Index Array(array=w252, index=w251) -> (element=w250:string)
        n175 = call <vilib>:"NT Write String.vi"("value"=w250, "name"="TestMode/TestName" ("Name")) -> ()  [unwired: 9 in, 1 out]
        n176 = property on="Progress" class="Clust (strict)"("Visible"=TRUE) -> ()  [unwired: 2 in, 2 out]
        n177 = property on="Motor" class="Clust (strict)"("Visible"=w247) -> ()  [unwired: 2 in, 2 out]
        n178 = property on="Test Slider" class="Slide (strict)"("Visible"=w247) -> ()  [unwired: 2 in, 2 out]
        n179 = property on="On/Off" class="Bool (strict)"("Visible"=w247) -> ()  [unwired: 2 in, 2 out]
        n180 = property on="Rev/Fwd" class="Clust (strict)"("Visible"=w247) -> ()  [unwired: 2 in, 2 out]
        n181 = property on="Test Ring" class="Ring (strict)"("Visible"=w247) -> ()  [unwired: 2 in, 2 out]
      }
      event "Select Auto": Mouse Enter {
        # "Populate the combo box with the list of autonomous options"
        n182 = event-data() -> ()  [unwired: 1 in, 1 out]
        n183 = call <vilib>:"NT Read String Array.vi"("name"="Auto List" ("Name")) -> ("value"=w254:string[])  [unwired: 8 in, 2 out]
        n184 = property on="Select Auto" class="CmbBox"("Strings[]"=w254) -> ()  [unwired: 2 in, 2 out]
      }
      event "Select Auto": Value Change {
        # "User modified the Auto Selection. Write to NT variable so robot knows."
        n185 = event-data() -> ("NewVal"=w256:string)  [unwired: 1 in]
        n186 = call <vilib>:"NT Write String.vi"("value"=w256, "name"="Auto Selector" ("Name")) -> ()  [unwired: 9 in, 1 out]
      }
      event "CheckList": Double Click {
        # "Shift clears all"
        # "Update symbols on the listbox"
        n187 = event-data() -> ("PlatMods.Shift"=w258:bool, "Row"=w260:i32)  [unwired: 1 in]
        n188 = case shown="True" w258 {
          tunnel: w260 -> [w264 _]
          tunnel: 1 -> [w263 _]
          frame False {
            n189 = property on="CheckList" class="LstBox (strict)"() -> ("Item Symbols"=w262:i32[])  [unwired: 2 in, 2 out]
            n190 = Replace Array Subset(array=w262, new element=w263, index=w264) -> (w261:i32[])
            n191 = property on="CheckList" class="LstBox (strict)"("Item Symbols"=w261) -> ()  [unwired: 2 in, 2 out]
          }
          frame True {
            w265 = 0 ("Top Row")
            n192 = property on="CheckList" class="LstBox (strict)"() -> ("Number of Rows"=w267:u32)  [unwired: 2 in, 2 out]
            n193 = Initialize Array(0, w267) -> (w266:i32[])
            n194 = property on="CheckList" class="LstBox (strict)"("Top Row"=w265, "Value"=w265, "Item Symbols"=w266) -> ()  [unwired: 2 in, 2 out]
          }
        }
      }
      event "CheckList": Key Down {
        # "Update symbols on the listbox\nLeft and right keys check and uncheck"
        n195 = event-data() -> ("VKey"=w270:T18)  [unwired: 1 in]
        n196 = case shown="\"Left\", \"Right\"" w270 {
          selector: w270 -> [w275 _]
          tunnel: eventvkey."Left" ("VKey") -> [w273 _]
          frame "Left", "Right" {
            n197 = Equal?(x=w273, y=w275) -> (x = y?=w274:bool)
            n198 = Select(t=0, s=w274, f=1) -> (s? t:f=w276:i32)
            n199 = property on="CheckList" class="LstBox (strict)"() -> ("Item Symbols"=w279:i32[])  [unwired: 2 in, 2 out]
            n200 = Replace Array Subset(array=w279, new element=w276, index="CheckList") -> (w278:i32[])
            n201 = property on="CheckList" class="LstBox (strict)"("Item Symbols"=w278) -> ()  [unwired: 2 in, 2 out]
          }
          frame Default {
          }
        }
      }
      event "Motor.Enable": Value Change {
        # "When the test mode otor enable helper is set, update that\ntree row item's value"
        n202 = event-data() -> ("NewVal"=w284:bool)  [unwired: 1 in]
        n203 = Unbundle("Motor") -> ("Value"=w283:dbl)  [unwired: 1 out]
        n204 = Select(t=w283, s=w284, f=0.0) -> (s? t:f=w281:dbl)
        n205 = call <vilib>:"NT Write Number.vi"("value"=w281, "name"=w280) -> ()  [unwired: 9 in, 1 out]
      }
      event "Test Slider": Value Change {
        # "When the test mode slider helper is set, update that\ntree row item's value"
        n206 = event-data() -> ("NewVal"=w286:dbl)  [unwired: 1 in]
        n207 = call <vilib>:"NT Write Number.vi"("value"=w286, "name"=w287) -> ()  [unwired: 9 in, 1 out]
      }
      event "On/Off": Value Change {
        # "When the test mode on/off helper value is set, update that\ntree row item's value"
        n208 = event-data() -> ("NewVal"=w290:bool)  [unwired: 1 in]
        n209 = Boolean To (0,1)(Boolean=w290) -> (0, 1=w289:i16)
        n210 = call <vilib>:"NT Write Number.vi"("value"=w289, "name"=w288) -> ()  [unwired: 9 in, 1 out]
      }
      event "Rev/Fwd": Value Change {
        # "When the test mode helper value for relays is set, update that\ntree row item's value"
        n211 = event-data() -> ("NewVal.Forward"=w297:bool, "NewVal.Reverse"=w296:bool)  [unwired: 1 in]
        n212 = Boolean To (0,1)(Boolean=w297) -> (0, 1=w293:i16)
        n213 = Boolean To (0,1)(Boolean=w296) -> (0, 1=w295:i16)
        n214 = Negate(x=w295) -> (-x=w294:i16)
        n215 = Add(x=w293, y=w294) -> (x+y=w292:i16)
        n216 = call <vilib>:"NT Write Number.vi"("value"=w292, "name"=w291) -> ()  [unwired: 9 in, 1 out]
      }
      event "Test Ring": Value Change {
        # "When a test mode helper value is selected from the ring,\nset the tree item's variable to the string value"
        n217 = event-data() -> ("NewVal"=w300:u16)  [unwired: 1 in]
        n218 = property on="Test Ring" class="Ring (strict)"() -> ("Strings []"=w301:string[])  [unwired: 2 in, 2 out]
        n219 = Index Array(array=w301, index=w300) -> (element=w299:string)
        n220 = call <vilib>:"NT Write String.vi"("value"=w299, "name"=w298) -> ()  [unwired: 9 in, 1 out]
      }
      event "Rec Mode": Value Change {
        # "Update globals for recording mode and path to read log from.\nClear when logging and let NetworkTables set path for vision to\nuse."
        n221 = event-data() -> ("NewVal"=w310:enum32{"Stop", "Record", "Playback"})  [unwired: 1 in]
        n222 = global write "WPI_DashboardLogging Global.vi" "Logging Filename"(path "") -> ()
        n223 = global write "WPI_DashboardLogging Global.vi" "Recording"(w310) -> ()
        n224 = case shown="\"Playback\"" w310 {
          tunnel: w309 -> [_ w312 w320]
          tunnel: [_ _ w319] -> w307
          tunnel: [_ _ w318] -> _
          tunnel: w305 -> [_ _ w316]
          tunnel: cluster{i32, i32} {-250, 170} -> [_ _ w315]
          tunnel: [_ _ T19 {"Image Size"=TRUE, "Image Type"=TRUE, "Pixel Value"=TRUE, "ROI Information"=TRUE, "Zoom Factor"=FALSE} ("Image Information Shown:All Elements")] -> w302
          tunnel: [_ _ TRUE ("Zoom Factor")] -> w303
          frame Default {
          }
          frame "Stop", "Record" {
            # "Place Window too"
            n225 = invoke class="VI" method="FP.Close"(reference=w312) -> (reference out=w311:refnum<vi>)  [unwired: 2 in, 2 out]
            n226 = invoke class="VI" method="Abort VI"(reference=w311) -> ()  [unwired: 2 in, 3 out]
          }
          frame "Playback" {
            n227 = call "Open Playback Panel.vi"("Offset"=w315, "DB VI Ref"=w316, "Playback in"=w320) -> ("Playback out"=w317:refnum<vi>)  [unwired: 8 in]
            n228 = register-events(w317) -> (reference out=w319:refnum<event-registration>, error out=w318:errorcluster)  [unwired: 2 in]
          }
        }
        n229 = property on="Camera Image" class="ImageControl"("Image Information Shown"=w302, "Image Information Visible"=w303) -> ()  [unwired: 2 in, 2 out]
        n230 = call <vilib>:"WPI_DashboardNT Log FieldName Cache.vi"("Operation"=enum16{"Lookup/Add", "Index", "Clear"}."Clear") -> ()  [unwired: 8 in, 3 out]
      }
      event Panel Close {
        w321 = enum32{"Stop", "Record", "Playback"}."Stop" ("Rec Mode")
        # "Playback window has been closed, abort"
        n231 = event-data() -> ()  [unwired: 1 in, 4 out]
        n232 = local write "Rec Mode"(w321) -> ()
        n233 = global write "WPI_DashboardLogging Global.vi" "Recording"(w321) -> ()
      }
      event Panel Close {
        # "Abort playback window and ourself"
        n234 = event-data() -> ()  [unwired: 1 in, 4 out]
        n235 = invoke class="VI" method="FP.Close"(reference=w324) -> (reference out=w323:refnum<vi>)  [unwired: 2 in, 2 out]
        n236 = invoke class="VI" method="Abort VI"(reference=w323) -> (error out=w322:errorcluster)  [unwired: 2 in, 2 out]
        n237 = invoke class="VI" method="Abort VI"(error in=w322) -> ()  [unwired: 2 in, 3 out]
      }
      event "Tree": Double Click {
        n238 = event-data() -> ("PlatMods"=w330:T21, "Tag"=w327:string)  [unwired: 1 in]
        n239 = Unbundle(w330) -> ("Shift"=w329:bool)  [unwired: 4 out]
        n240 = String Subset(string=w327, length (rest)=1 ("length (rest)")) -> (substring=w326:string)  [unwired: 1 in]
        n241 = Not(x=w329) -> (.not. x?=w328:bool)
        n242 = case shown="\"/\"" w326 {
          tunnel: w327 -> [_ w332]
          tunnel: w328 -> [_ w331]
          frame Default {
          }
          frame "/" {
            n243 = call <vilib>:"NT Update Persistence.vi"("Persistence"=w331, "Name"=w332) -> ()  [unwired: 9 in, 1 out]
          }
        }
      }
    }
  }
  n244 = while {
    tunnel: w53 -> [w334]
    i -> [w337]
    stop <- FALSE stop-if-true
    n245 = Wait (ms)(milliseconds to wait=u32 100) -> ()  [unwired: 1 out]
    n246 = case shown="\"Playback\"" "Rec Mode" {
      tunnel: w337 -> [_ _ w352]
      tunnel: [u32 2829099 ("Base Color") u32 11141120 ("Target Color") w341] -> w333
      frame "Stop", Default {
        # "Reset the color, extra updates don't cost much"
      }
      frame "Record" {
      }
      frame "Playback" {
        # "Playback"
        n247 = Quotient & Remainder(x=w352, y=u32 50 ("milliseconds to wait")) -> (x-y*floor(x/y)=w348:u32)  [unwired: 1 out]
        n248 = Divide(x=w348, y=u32 50 ("milliseconds to wait")) -> (x/y=w345:dbl)
        n249 = Multiply(x=6.283185307179586, y=w345) -> (x*y=w350:dbl)
        n250 = Sine(x=w350) -> (sin(x)=w349:dbl)
        n251 = Absolute Value(x=w349) -> (abs(x)=w342:dbl)
        n252 = call "Interpolate RGB Color.vi"("Proportion"=w342, "Target Color"=u32 30976, "Base Color"=u32 2829099) -> ("Result Color"=w341:u32)  [unwired: 8 in]
      }
    }
    n253 = property class="Pane"(reference=w334, "PaneColor"=w333) -> ()  [unwired: 1 in, 2 out]
  }
  n254 = local write "Dashboard Tab"(T3."Main" ("Dashboard Tab")) -> ()
  n255 = property on="On/Off" class="Bool (strict)"("Visible"=w28) -> ()  [unwired: 2 in, 2 out]
  n256 = property on="Motor" class="Clust (strict)"("Visible"=w28) -> ()  [unwired: 2 in, 2 out]
  n257 = property on="Progress" class="Clust (strict)"("Visible"=w28) -> ()  [unwired: 2 in, 2 out]
  n258 = property on="Test Ring" class="Ring (strict)"("Visible"=w28) -> ()  [unwired: 2 in, 2 out]
  n259 = property on="Rev/Fwd" class="Clust (strict)"("Visible"=w28) -> ()  [unwired: 2 in, 2 out]
  n260 = while {
    tunnel: u16 1741 ("timeout ms (25000)") -> [w354]
    stop <- FALSE stop-if-true
    n261 = TCP Create Listener(10:w354) -> (0:w353:errorcluster, 3:w355:refnum<k5>)  [unwired: 4 in, 1 out]
    n262 = case shown="No Error" w353 {
      selector: w353 -> [w357 _]
      tunnel: w355 -> [w358 _]
      frame No Error {
        n263 = while {
          tunnel: w358 -> [w361]
          tunnel: w357 -> [w360]
          stop <- FALSE stop-if-true
          n264 = TCP Wait On Listener(8:w360, 11:w361) -> (0:w362:errorcluster, 4:w363:refnum<k5>)  [unwired: 2 in, 3 out]
          n265 = local write "TCP"(w363) -> ()
          n266 = case shown="Error" w362 {
            frame No Error {
            }
            frame Error {
              n267 = Wait (ms)(milliseconds to wait=u32 1000) -> ()  [unwired: 1 out]
            }
          }
        }
      }
      frame Error {
        n268 = Wait (ms)(milliseconds to wait=u32 1000) -> ()  [unwired: 1 out]
      }
    }
  }
  n269 = global write "WPI_DashboardLogging Global.vi" "Recording"(w48) -> ()
  n270 = local write "Rec Mode"(w48) -> ()
  n271 = call <vilib>:"NT Write String.vi"("value"="Select Auto", "name"="Auto Selector" ("Name")) -> ()  [unwired: 9 in, 1 out]
  n272 = control-ref of="Field Picture"() -> (w11:refnum<vi>)
  n273 = control-ref of="ROBOT"() -> (w13:refnum<vi>)
  n274 = control-ref of="Field Picture"() -> (w14:refnum<vi>)
  n275 = call <vilib>:"FieldDisp_Element_Prepare.vi"("Element File Name"="Robot_kitbot_5.png" ("Picture FIle Name"), "Element Picture Ref"=w13, "Field Picture Ref"=w14) -> ("Field Element Info"=w6:T22)  [unwired: 7 in, 1 out]
  n276 = call <vilib>:"FieldDisp_Field_Disp.vi"("Field Selector"="2023 Charged Up", "Picture in"=w11) -> ("error out"=w9:errorcluster)  [unwired: 9 in]
  n277 = while {
    stop <- FALSE stop-if-true
    n278 = call-poly <vilib>:"NT Write Value.vi"("value"="DONUT PRESS", "name"="zKALINDASTUFF/DONUT" ("Name")) -> ()  [unwired: 9 in, 1 out]
    n279 = call "Banana.vi"("Boolean"="DONUT PRESS") -> ("Boolean 2"=→"Bananas Engaged":bool)  [unwired: 10 in]
  }
  n280 = disable-structure shown="Disabled" {
    frame Disabled {
      n281 = while {
        stop <- FALSE stop-if-true
        n282 = call-poly <vilib>:"NT Write Value.vi"("value"="Dont Question it", "name"="zKALINDASTUFF/POPCORN" ("Name")) -> ()  [unwired: 9 in, 1 out]
        n283 = call "Popcorn.vi"("Boolean"="Dont Question it") -> ("Boolean 2"=→"Popcorn Engaged":bool)  [unwired: 10 in]
      }
    }
    frame Enabled {
    }
  }
  n284 = call "OpenCV_LabVIEW_HueConvert.vi"() -> ("OpenCV to LV"=w4:dbl, "LV to OpenCV"=w5:dbl)  [unwired: 10 in]
  n285 = while {
    tunnel: [w385] -> _
    tunnel: w27 -> [w377]
    tunnel: w9 -> [_]
    tunnel: w6 -> [w376]
    tunnel: w5 -> [w375]
    tunnel: w4 -> [w374]
    i -> [w385]
    stop <- FALSE stop-if-true
    n286 = call <vilib>:"WPI_DashboardRetrieveStatusInfo.vi"("Window Mode Notifier"=w377, "TCP Cnx"="TCP") -> ("Power and Errors"=w380:T24, "Robot Metrics"=w383:T25, "Status Info"=w384:T26, "Control Info"=w381:T27, "Robot Mode"=w379:T4, "Process?"=w382:bool)  [unwired: 4 in]
    "Mode" <- w379
    n287 = case shown="True" w382 {
      tunnel: w384 -> [_ w493]
      tunnel: w383 -> [_ w492]
      tunnel: w381 -> [_ w491]
      tunnel: w380 -> [_ w490]
      tunnel: w379 -> [_ _]
      tunnel: w376 -> [_ w480]
      tunnel: w375 -> [_ w453]
      tunnel: w374 -> [_ w452]
      frame False {
        n288 = Wait (ms)(milliseconds to wait=u32 20) -> ()  [unwired: 1 out]
      }
      frame True {
        w422 = 9.0 ("y")
        # "The 2022 version had some\ncustom stuff here that didn't \nmake much sense...."
        # "swap motors to match\ncharts and include battery"
        # "HIT WALL WARNING"
        # "MAIN"
        # "Debug - Right Speed"
        # "Debug - Left Speed"
        # "Debug - Camera Tab"
        # "Shooter Tab"
        # "tab changed."
        # "y"
        # "x"
        n289 = Unbundle By Name(w492) -> ()  [unwired: 1 out]
        n290 = Unbundle By Name(w490) -> ("Robot IP"=→"Robot IP":string)
        n291 = Unbundle By Name(w493) -> ()  [unwired: 2 out]
        n292 = Unbundle By Name(w491) -> ("Joystick Values"=w489:T28)  [unwired: 1 out]
        n293 = Index Array(array=w489) -> (element #1=w488:T29, element #2=w487:T29)  [unwired: 2 in]
        n294 = call "Prepare Joystick Data for Displays.vi"("Joystick Values"=w487) -> ("Buttons"=→"JS2 Buttons":T30, "Z Axis"=→"JS2 Z":dbl, "Cartesian Data"=→"JS2 Graph":cluster{"X axis":dbl, "X axis":dbl}[])  [unwired: 8 in]
        n295 = call "Prepare Joystick Data for Displays.vi"("Joystick Values"=w488) -> ("Buttons"=→"JS1 Buttons":T30, "Z Axis"=→"JS1 Z":dbl, "Cartesian Data"=→"JS1 Graph":cluster{"X axis":dbl, "X axis":dbl}[])  [unwired: 8 in]
        n296 = call-poly <vilib>:"NT Read Value.vi"("name"="Vision/Left vision found count") -> ("value"=w470:dbl)  [unwired: 8 in, 2 out]
        n297 = call-poly <vilib>:"NT Read Value.vi"("name"="Vision/Right vision found count") -> ("value"=w466:dbl)  [unwired: 8 in, 2 out]
        n298 = feedback-in #1(w470) -> ()
        n299 = feedback #1() -> (w469:dbl)  [unwired: 1 in]
        n300 = feedback #2() -> (w465:dbl)  [unwired: 1 in]
        n301 = feedback-in #2(w466) -> ()
        n302 = call-poly <vilib>:"NT Read Value.vi"("name"="Vision/Left vision connect") -> ("value"=→"Left Cam Connected":bool)  [unwired: 8 in, 2 out]
        n303 = call-poly <vilib>:"NT Read Value.vi"("name"="Vision/Right vision connect") -> ("value"=→"Right Cam Connected":bool)  [unwired: 8 in, 2 out]
        n304 = Not Equal?(x=w470, y=w469) -> (x != y?=→"Left April Tag Updated":bool)
        n305 = Not Equal?(x=w466, y=w465) -> (x != y?=→"Right April Tag Updated":bool)
        n306 = call-poly <vilib>:"NT Read Value.vi"("name"="Vision/Xcurrent in feet") -> ("value"=w478:dbl)  [unwired: 8 in, 2 out]
        "Odom X Pos Ft" <- w478
        n307 = call-poly <vilib>:"NT Read Value.vi"("name"="Vision/Y current in feet") -> ("value"=w462:dbl)  [unwired: 8 in, 2 out]
        "Odom Y Pos Ft" <- w462
        n308 = call-poly <vilib>:"NT Read Value.vi"("name"="Vision/angle current") -> ("value"=w463:dbl)  [unwired: 8 in, 2 out]
        "Odom Heading Deg" <- w463
        n309 = local read "Dashboard Tab"() -> (w459:T3)
        n310 = call <vilib>:"Conv_Feet_Meters.vi"("Feet"=w478) -> ("Meters"=w477:dbl)  [unwired: 10 in]
        n311 = call <vilib>:"Conv_Feet_Meters.vi"("Feet"=w462) -> ("Meters"=w476:dbl)  [unwired: 10 in]
        n312 = call <vilib>:"Conv_Deg_Radians.vi"("Degress"=w463) -> ("Radians"=w479:dbl)  [unwired: 10 in]
        n313 = Equal?(x=T23."Field" ("Dashboard Tab"), y=w459) -> (x = y?=w461:bool)
        n314 = feedback-in #3(w459) -> ()
        n315 = feedback #3() -> (w458:T3)  [unwired: 1 in]
        n316 = Not Equal?(x=w459, y=w458) -> (x != y?=w457:bool)
        n317 = case shown="True" w461 {
          tunnel: w480 -> [w497 w502]
          tunnel: w479 -> [_ w505]
          tunnel: w477 -> [_ w504]
          tunnel: w476 -> [_ w503]
          tunnel: w457 -> [w496 w501]
          frame False {
            n318 = case shown="True" w496 {
              tunnel: w497 -> [_ w498]
              frame False {
              }
              frame True {
                n319 = Unbundle By Name(w498) -> ("Element Picture Ref"=w499:refnum<vi>)
                n320 = property class="Pict"(reference=w499, "Visible"=FALSE) -> ()  [unwired: 1 in, 2 out]
              }
            }
          }
          frame True {
            # "Update display\nof field element\n(robot)"
            n321 = call <vilib>:"Pose2d_New.vi"("Heading"=w505, "Y"=w503, "X"=w504) -> ("out POSe"=w506:T31)  [unwired: 8 in]
            n322 = call <vilib>:"FieldDisp_Element_Disp.vi"("Element Pose"=w506, "Element Info"=w502) -> ()  [unwired: 10 in]
            n323 = case shown="True" w501 {
              tunnel: w502 -> [_ w507]
              frame False {
              }
              frame True {
                n324 = Unbundle By Name(w507) -> ("Element Picture Ref"=w508:refnum<vi>)
                n325 = property class="Pict"(reference=w508, "Visible"=TRUE) -> ()  [unwired: 1 in, 2 out]
              }
            }
          }
        }
        n326 = call-poly <vilib>:"NT Read Value.vi"("name"="Auto/SelectedAuto") -> ("value"=→"Selected Auto":string)  [unwired: 8 in, 2 out]
        n327 = call-poly <vilib>:"NT Read Value.vi"("name"="Encoder 2(Left) Speed" ("Name")) -> ("value"=w396:dbl)  [unwired: 8 in, 2 out]
        "Left Speed" <- w396
        n328 = call-poly <vilib>:"NT Read Value.vi"("name"="LeftSpeedDemand" ("Name")) -> ("value"=w397:dbl)  [unwired: 8 in, 2 out]
        "Left Speed Demand" <- w397
        n329 = call-poly <vilib>:"NT Read Value.vi"("name"="Encoder 1(Right) Speed" ("Name")) -> ("value"=w398:dbl)  [unwired: 8 in, 2 out]
        "Right Speed" <- w398
        n330 = call-poly <vilib>:"NT Read Value.vi"("name"="RigthSpeedDemand" ("Name")) -> ("value"=w399:dbl)  [unwired: 8 in, 2 out]
        "Right Speed Demand" <- w399
        n331 = call-poly <vilib>:"NT Read Value.vi"("name"="LidarDistance") -> ("value"=w420:dbl)  [unwired: 8 in, 2 out]
        "Lidar" <- w420
        n332 = call "Format-shooter-speed-mode.vi"() -> ("Shooter Speed Mode Color"=w410:u32, "Shooter Speed Mode Text"=→"To infinity and beyond?":string)  [unwired: 10 in]
        n333 = call-poly <vilib>:"NT Read Value.vi"("name"="RobotDrive Motors" ("Name")) -> ("value"=w400:dbl[])  [unwired: 8 in, 2 out]
        n334 = Bundle("value"=w399, "value"=w398) -> (→"Speed Chart Right":cluster{"value":dbl, "value":dbl})  [unwired: 1 in]
        n335 = Bundle("value"=w397, "value"=w396) -> (→"Speed Chart Left":cluster{"value":dbl, "value":dbl})  [unwired: 1 in]
        n336 = Greater?(x=w399, y=w422) -> (0:w426:bool)
        n337 = Greater?(x=w397, y=w422) -> (0:w427:bool)
        n338 = Index Array(array=w400, index #1=1, index #4=0) -> (element #1=w405:dbl, element #2=w406:dbl, element #3=w404:dbl, element #4=w409:dbl)  [unwired: 2 in]
        n339 = call-poly <vilib>:"NT Read Value.vi"("name"="Reverse?") -> ("value"=→"Reverse":bool)  [unwired: 8 in, 2 out]
        n340 = call-poly <vilib>:"NT Read Value.vi"("name"="ClimbOverride" ("Name")) -> ("value"=→"Climb Override":bool)  [unwired: 8 in, 2 out]
        n341 = call-poly <vilib>:"NT Read Value.vi"("name"="ClimbState" ("Name")) -> ("value"=→"Climbing Stages":dbl)  [unwired: 8 in, 2 out]
        n342 = property on="To infinity and beyond?" class="Str"("Text.BG Color"=w410, "Text.FG Color"=w410, "Text.BGColor"=w410) -> ()  [unwired: 2 in, 2 out]
        n343 = call-poly <vilib>:"NT Read Value.vi"("name"="DriveMode" ("Name")) -> ("value"=→"Drive Mode":string)  [unwired: 8 in, 2 out]
        n344 = Less?(x=w420, y=4.0) -> (x < y?=w425:bool)
        n345 = Or(x=w427, y=w426) -> (x .or. y?=w424:bool)
        n346 = call-poly <vilib>:"NT Write Value.vi"("value"="ARE YOU READY TO RUMBLE", "name"="RumbleToggle" ("Name")) -> ()  [unwired: 9 in, 1 out]
        n347 = Bundle("Numeric"=w404, "Numeric"=w405) -> (→"MotorChart R" →"MotorSliders R":cluster{"Numeric":dbl, "Numeric":dbl})  [unwired: 1 in]
        n348 = Bundle("Numeric"=w406, "Numeric"=w409) -> (→"MotorChart L" →"MotorSliders L":cluster{"Numeric":dbl, "Numeric":dbl})  [unwired: 1 in]
        n349 = And(x=w424, y=w425) -> (x .and. y?=→"Wall!":bool)
        n350 = call-poly <vilib>:"NT Read Value.vi"("name"="/vision/deviationThreshold" ("Name")) -> ("value"=→"Deviation Threshold 2":dbl)  [unwired: 8 in, 2 out]
        n351 = call-poly <vilib>:"NT Write Value.vi"("value"="Deviation Threshold", "name"="/vision/deviationThreshold" ("Name")) -> ()  [unwired: 9 in, 1 out]
        n352 = local read "Current Filter"() -> (w454:T8)
        n353 = case shown="True" "Update\nVision\nTuning" {
          tunnel: w453 -> [_ w495]
          frame False {
          }
          frame True {
            n354 = local read "New Filter"() -> (w494:T8)
            n355 = call "Update_Vision_Tuning.vi"("New Filter"=w494, "LV to OpenCV"=w495) -> ()  [unwired: 10 in]
          }
        }
        n356 = call-poly <vilib>:"NT Read Value.vi"("name"="ShooterRPM" ("Name")) -> ("value"=w443:dbl)  [unwired: 8 in, 2 out]
        "Shooter Speed" <- w443
        n357 = call-poly <vilib>:"NT Read Value.vi"("name"="/vision/filterHeight" ("Name")) -> ("value"=→"Filter Height 2":dbl)  [unwired: 8 in, 2 out]
        n358 = call-poly <vilib>:"NT Read Value.vi"("name"="ShooterMotorOutput" ("Name")) -> ("value"=w441:dbl)  [unwired: 8 in, 2 out]
        "Motor Output" <- w441
        n359 = call "read_current_vision_tuning.vi"("OpenCV to LV"=w452, "Current Filter in"=w454) -> ("Current Filter out"=→"Current Filter":T8)  [unwired: 9 in]
        n360 = call-poly <vilib>:"NT Read Value.vi"("name"="ShooterSpeedDemand" ("Name")) -> ("value"=→"Target Shooter Speed":dbl)  [unwired: 8 in, 2 out]
        n361 = Bundle("Shooter Demand"="Shooter Demand", "value"=w443, "value"=w441) -> (→"Shooter Speed Trend":T34)  [unwired: 1 in]
        n362 = call-poly <vilib>:"NT Write Value.vi"("value"="Filter Height", "name"="/vision/filterHeight" ("Name")) -> ()  [unwired: 9 in, 1 out]
        n363 = call-poly <vilib>:"NT Write Value.vi"("value"="Shooter Demand", "name"="ShooterSpeedRequest" ("Name")) -> ()  [unwired: 9 in, 1 out]
      }
    }
  }
